vi "Normal Drive (Autonomous).vi"(1 "Execute":bool=TRUE, 2 "Distance (Feet)":dbl=10.0, 3 "Percent Speed":dbl=0.8) -> (4 "Done Executing":bool)   [LabVIEW 2012]
uses:
  Globals/Autonomous Joystick Emulation.vi
  Globals/Encoders Global.vi
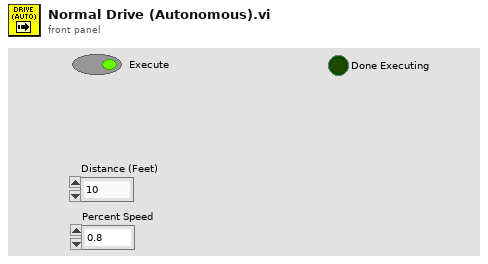
[diagram p1: front panel]
types:
  T1 = typedef "WPI_EncoderDevRef.ctl" = cluster{"DevStatus":errorcluster, "EncoderIndex":T2, "CounterIndex":T3, "DistancePerCount":dbl, "Decoding Type":T4}
  T2 = typedef "FPGA_EncoderIdx.ctl" = enum8{"Enc 0", "Enc 1", "Enc 2", "Enc 3", "Invalid"}
  T3 = typedef "FPGA_CounterCtrSystemIndex.ctl" = enum8{"Ctr 0", "Ctr 1", "Ctr 2", "Ctr 3", "Ctr 4", "Ctr 5", "Ctr 6", "Ctr 7", "Invalid"}
  T4 = typedef "WPI_EncoderType.ctl" = enum16{"1x", "2x", "4x"}
  T5 = cluster{"Front Left":T1, "Front Right":T1, "Rear Left":T1, "Rear Right":T1, "Shooter":T1}
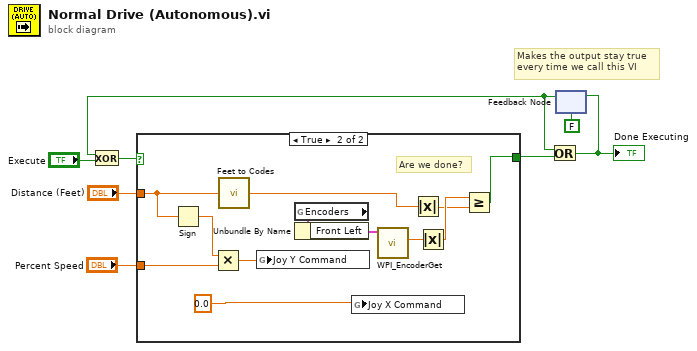
[diagram p0: block diagram]
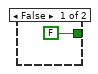
[diagram p2: hidden frame]
diagram:
  # "Makes the output stay true\nevery time we call this VI"
  n1 = feedback #1(FALSE) -> (w3:bool)
  n2 = Exclusive Or(1:"Execute", 2:w3) -> (0:w8:bool)
  n3 = case shown="True" w8 {
    tunnel: [FALSE w21] -> w6
    tunnel: "Percent Speed" -> [_ w16]
    tunnel: "Distance (Feet)" -> [_ w15]
    frame False {
    }
    frame True {
      # "Are we done?"
      n4 = Sign(1:w15) -> (0:w14:dbl)
      n5 = Multiply(x=w14, y=w16) -> (x*y=w11:dbl)
      n6 = call "Feet to Codes.vi"("Feet"=w15) -> ("Codes"=w20:dbl)
      n7 = global write "Autonomous Joystick Emulation.vi" "Joy Y Command"(w11) -> ()
      n8 = global read "Encoders Global.vi" "Encoders"() -> (w19:T5)
      n9 = Unbundle By Name(w19) -> ("Front Left"=w18:T1)
      n10 = global write "Autonomous Joystick Emulation.vi" "Joy X Command"(0.0 ("Joy X Command")) -> ()
      n11 = call <vilib>:"WPI_EncoderGet.vi"("EncoderDevRef"=w18) -> ("Distance"=w17:dbl)  [unwired: 5 in, 5 out]
      n12 = Absolute Value(x=w20) -> (abs(x)=w12:dbl)
      n13 = Absolute Value(x=w17) -> (abs(x)=w13:dbl)
      n14 = Greater Or Equal?(x=w13, y=w12) -> (x >= y?=w21:bool)
    }
  }
  n15 = Or(x=w3, y=w6) -> (x .or. y?=w2:bool)
  "Done Executing" <- w2
  n16 = feedback-in #1(w2) -> ()
